vi "JitterDACADC.vi"() -> ()   [LabVIEW 2009]
uses:
  <vilib>/Analysis/4window.llb/windowTd.ctl
  <vilib>/measure/maspectr.llb/FFT Power Spectrum for 1 Chan.vi
  <vilib>/Analysis/2dsp.llb/Resample (constant to constant,single -channel).vi
  <vilib>/ptbypt/NI_PtbyPt.lvlib
  <vilib>/Analysis/NI_AALBase.lvlib
  <vilib>/Analysis/NI_AALPro.lvlib
  <vilib>/measure/NI_MAPro.lvlib
panel:
  in  "Clock RMS time jitter":dbl format="%#_6p"
  in  "Sampling Rate":dbl=3000000.0 format="%#_6p"
  out "df":dbl
  out "averages completed":dbl=20.0
  out "DAC / ADC Sampling Period":dbl format="%#_6p"
  out "Elapsed Time (Seconds)":dbl
  in  "averaging parameters":T1={"averaging mode"=enum."RMS averaging", "weighting mode"=enum."Exponential", "number of averages"=20} {"number of averages" min=1}
  in  "Test System\n AWGN noise (dBm)":dbl=-180.0 format="%#.6f"
  out "Power Spectrum of sampled signal":cluster{"f0":dbl, "df":dbl, "magnitude":dbl[]}(graph)={"f0"=0.0, "df"=5000.0, "magnitude"=[]}
  out "Time Domain of Sampled Signal":waveform(dbl)(graph)={"t0"=timestamp(0 s since 1904-01-01), "dt"=3.3333333333333335e-07, "Y"=[]}
  in  "Duration (Seconds)":dbl=0.0002 min=0.0 format="%#_6e"
  in  "Tone Power (dBm)":dbl format="%#.6f"
  in  "Tone Frequency":dbl=750000.0 min=0.0 max=1000000000.0 format="%#.6p"
  in  "DAC clock RMS time jitter":dbl=1e-09 min=0.0 format="%#_6p"
  # "DAC/ADC Demo"
  # "Sampling Rate of tone fed into zero order\nhold DAC (also rate at which ADC samples).\nMust be > 2 * Tone Frequency"
  # "Jittery output from ADC Bonus Question: \nWhat is the SNR of this signal for no jitter?"
  # "Clue: It isn't tone power / System AWGN noise power. \nConsider bandwidth."
  # "Test System ADC"
  # "df ~= 1 / duration"
  # "Hz / Bin"
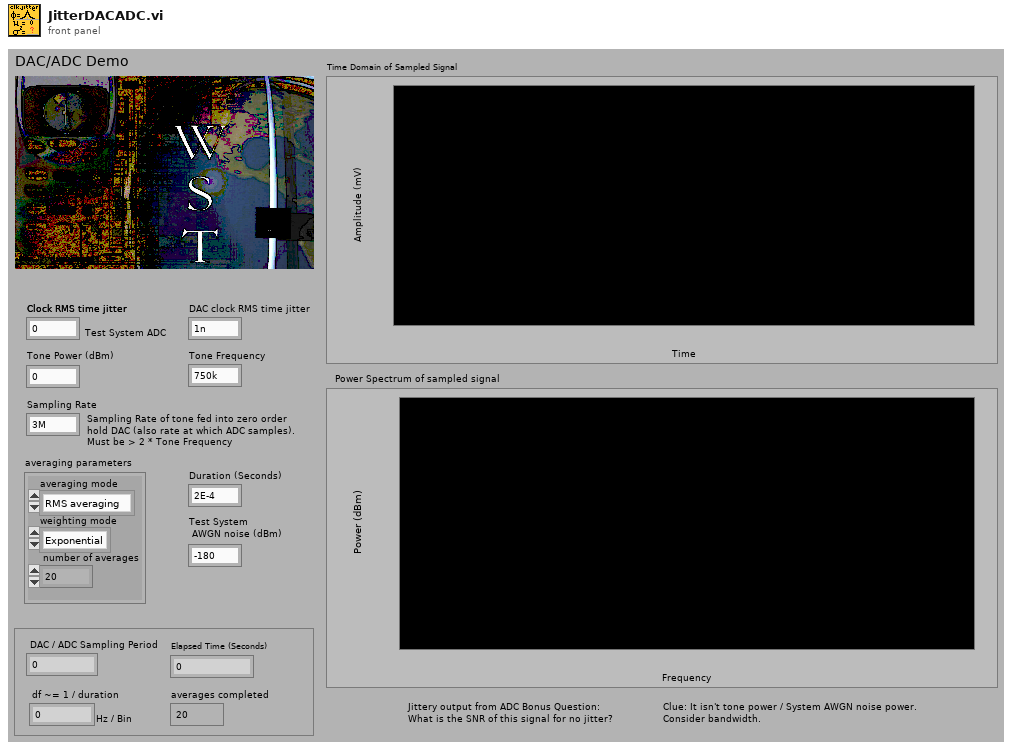
[diagram p1: front panel]
types:
  T1 = cluster{"averaging mode":enum16{"No averaging", "Vector averaging", "RMS averaging", "Peak hold"}, "weighting mode":enum16{"Linear", "Exponential"}, "number of averages":u32}
  T2 = typedef "NI_AALPro.lvlib/windowTd.ctl" = u32
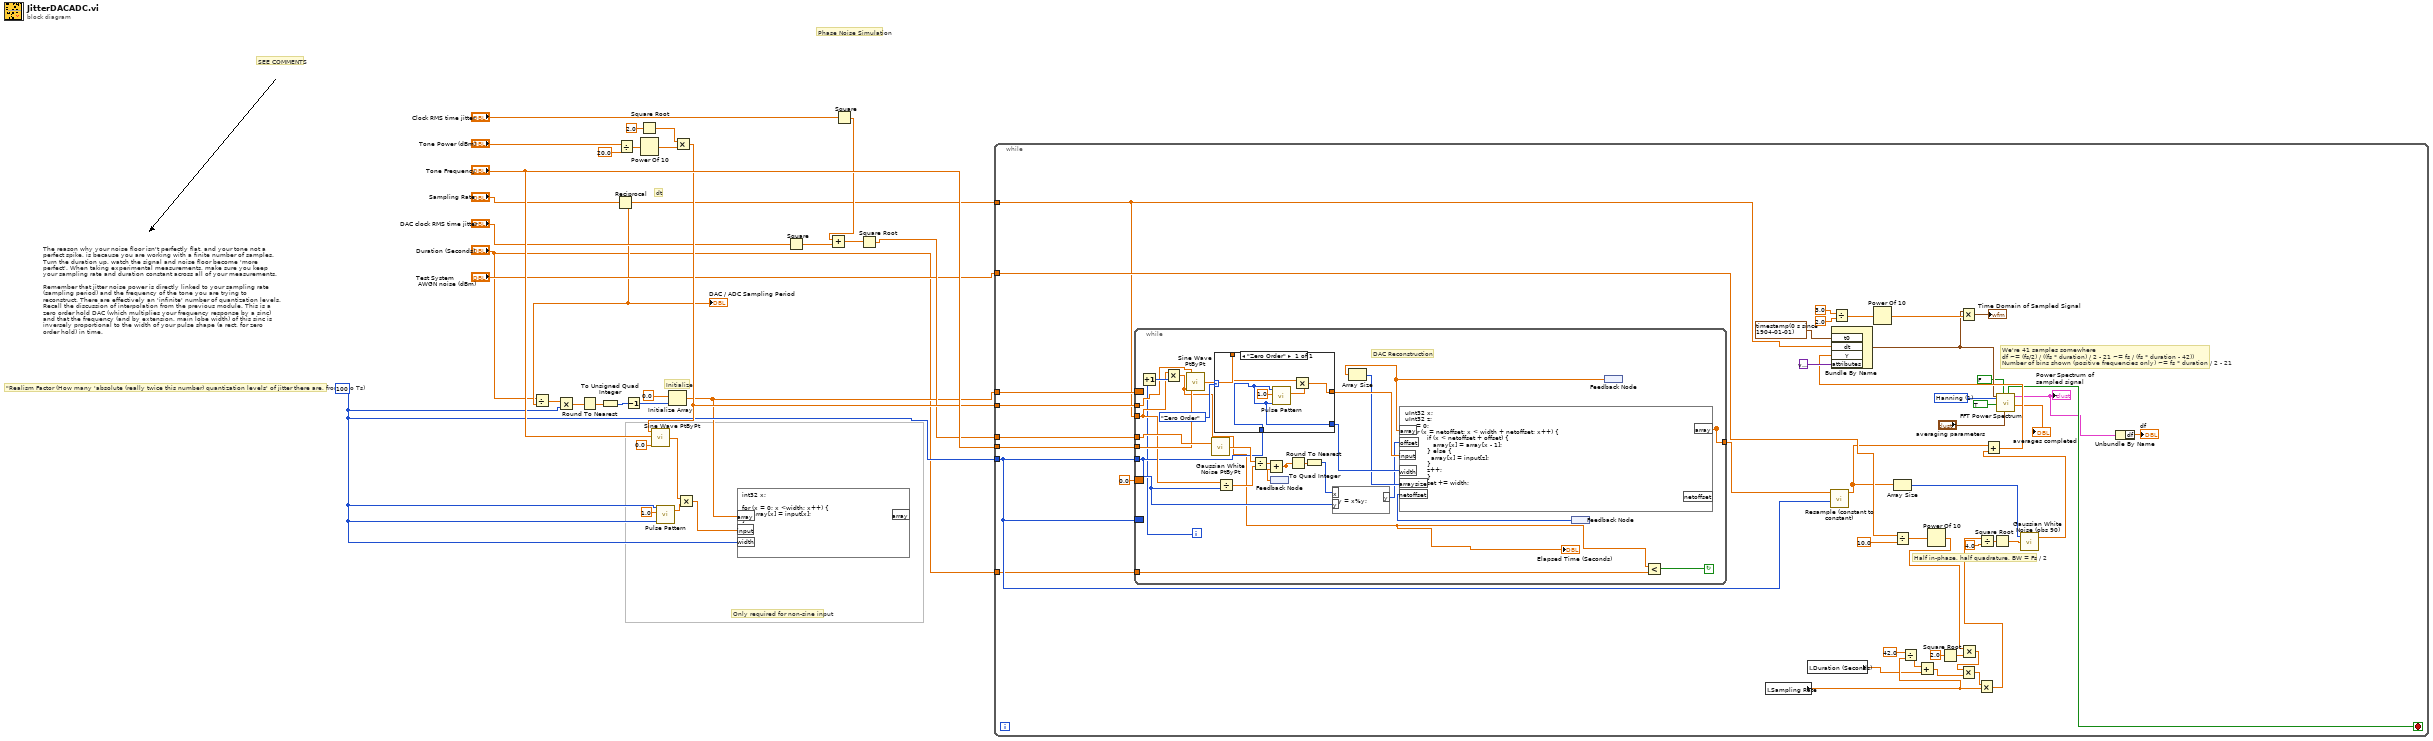
[diagram p0: block diagram]
diagram:
  w4 = 100
  # "SEE COMMENTS"
  # "The reason why your noise floor isn't perfectly flat, and your tone not a perfect spike, is because you are working with a finite number of samples. Turn the duration up, watch the signal and noise floor become 'more perfect'. When taking experimental measurements, make sure you keep your sampling rate and duration constant across all of your measurements.\n\nRemember that jitter noise power is directly linked to your sampling rate (sampling period) and the frequency of the tone you are trying to reconstruct. There are effectively an 'infinite' number of quantization levels. Recall the discussion of interpolation from the previous module. This is a zero order hold DAC (which multiplies your frequency response by a sinc) and that the frequency (and by extension, main lobe width) of this sinc is inversely proportional to the width of your pulse shape (a rect, for zero order hold) in time."
  # "Only required for non-sine input"
  # "\"Realism Factor (How many 'absolute (really twice this number) quantization levels' of jitter there are, from 0 to Ts)"
  # "Initialize"
  # "dt"
  # "Phase Noise Simulation"
  n1 = Reciprocal(x="Sampling Rate") -> (1/x=w5:dbl)
  "DAC / ADC Sampling Period" <- w5
  n2 = Divide(x="Duration (Seconds)", y=w5) -> (x/y=w21:dbl)
  n3 = Multiply(x=w21, y=w4) -> (x*y=w22:dbl)
  n4 = Round To Nearest(number=w22) -> (nearest integer value=w24:dbl)
  n5 = To Unsigned Quad Integer(1:w24) -> (0:w23:u64)
  n6 = Divide(x="Tone Power (dBm)", y=20.0) -> (x/y=w29:dbl)
  n7 = Decrement(x=w23) -> (x-1=w25:u64)
  n8 = Square Root(x=2.0) -> (sqrt(x)=w26:dbl)
  n9 = Power Of 10(x=w29) -> (10^x=w28:dbl)
  n10 = call <vilib>:"Pulse Pattern.vi"("width"=w4, "amplitude"=1.0, "samples"=w4) -> ("Pulse Pattern"=w15:dbl[])  [unwired: 1 in, 1 out]
  n11 = Initialize Array(0.0 ("element"), w25) -> (w2:dbl[])
  n12 = Multiply(x=w26, y=w28) -> (x*y=w18:dbl)
  n13 = call <vilib>:"Sine Wave PtByPt.vi"("time"=0.0, "frequency"="Tone Frequency", "amplitude"=w18) -> ("sine wave"=w13:dbl)  [unwired: 1 in]
  n14 = Multiply(x=w13, y=w15) -> (x*y=w14:dbl[])
  n15 = formula code="int32 x;\n\nfor (x = 0; x <width; x++) {\n     array[x] = input[x];\n}"("array"=w2, "input"=w14, "width"=w4) -> ()  [unwired: 1 out]
  n16 = Square(x="DAC clock RMS time jitter") -> (x^2=w11:dbl)
  n17 = Square(x="Clock RMS time jitter") -> (x^2=w10:dbl)
  n18 = Add(x=w10, y=w11) -> (x+y=w9:dbl)
  n19 = Square Root(x=w9) -> (sqrt(x)=w8:dbl)
  n20 = while {
    tunnel: "Tone Frequency" -> [w77]
    tunnel: w18 -> [w76]
    tunnel: w2 -> [w75]
    tunnel: w8 -> [w73]
    tunnel: "Test System\n AWGN noise (dBm)" -> [w66]
    tunnel: w5 -> [w60]
    tunnel: w4 -> [w52]
    tunnel: "Duration (Seconds)" -> [w38]
    stop <- w44 stop-if-true
    w59 = T2 1 items=["Rectangle"=0, "Hanning"=1, "Hamming"=2, "Blackman-Harris"=3, "Exact Blackman"=4, "Blackman"=5, "Flat Top"=6, "4 Term B-Harris "=7, "7 Term B-Harris"=8, "Low Sidelobe"=9, "Blackman Nuttall"=11, "Triangle"=30, "Kaiser"=60, "Dolph-Chebyshev"=61, "Gaussian"=62] ("window")
    # "We're 41 samples somewhere\ndf ~= (fs/2) / ((fs * duration) / 2 - 21 ~= fs / (fs * duration - 42))\nNumber of bins shown (positive frequencies only) ~= fs * duration / 2 - 21"
    # "Half in-phase, half quadrature, BW = Fs / 2"
    n21 = while {
      tunnel: w73 -> [w102]
      tunnel: w60 -> [w91]
      tunnel: w77 -> [w97]
      tunnel: w76 -> [w98]
      tunnel: w52 -> [w85]
      tunnel: [w89] -> w67
      tunnel: w38 -> [w80]
      border: w75 -> [_]
      border: w52 -> [_]
      border: 0.0 -> [_]
      i -> [w79]
      stop <- w104 continue-if-true
      # "DAC Reconstruction"
      n22 = Increment(x=w79) -> (x+1=w99:i32)
      n23 = Multiply(x=w91, y=w99) -> (x*y=w78:dbl)
      "Elapsed Time (Seconds)" <- w78
      n24 = call <vilib>:"Sine Wave PtByPt.vi"("time"=w78, "frequency"=w97, "amplitude"=w98) -> ("sine wave"=w103:dbl)  [unwired: 1 in]
      n25 = call <vilib>:"Gaussian White Noise PtByPt.vi"("standard deviation"=w102) -> ("Gaussian white noise"=w92:dbl)  [unwired: 2 in]
      n26 = case shown="\"Zero Order\"" enum16{"Zero Order"}."Zero Order" ("DAC Interpolation type") {
        tunnel: w85 -> [w105]
        tunnel: w103 -> [w107]
        tunnel: [w106] -> w101
        tunnel: [w105] -> w100
        frame "Zero Order" {
          n27 = call <vilib>:"Pulse Pattern.vi"("width"=w105, "amplitude"=1.0, "samples"=w105) -> ("Pulse Pattern"=w108:dbl[])  [unwired: 1 in, 1 out]
          n28 = Multiply(x=w107, y=w108) -> (x*y=w106:dbl[])
        }
      }
      n29 = Divide(x=w91, y=w85) -> (x/y=w93:dbl)
      n30 = Divide(x=w92, y=w93) -> (x/y=w83:dbl)
      n31 = feedback #1() -> (w82:dbl)
      n32 = Add(x=w83, y=w82) -> (x+y=w81:dbl)
      n33 = Round To Nearest(number=w81) -> (nearest integer value=w84:dbl)
      n34 = To Quad Integer(1:w84) -> (0:w87:i64)
      n35 = formula code="y = x%y;"("x"=w87, "y"=w85) -> ("y"=w86:i32)
      n36 = feedback #2() -> (w95:i32)
      n37 = feedback #3() -> (w90:dbl[])
      n38 = Array Size(array=w90) -> (size(s)=w94:i32)
      n39 = formula code="uInt32 x;\nuInt32 z;\n   z = 0;\n   for (x = netoffset; x < width + netoffset; x++) {\n           if (x < netoffset + offset) {\n              array[x] = array[x - 1];\n           } else {\n             array[x] = input[z];\n           }\n           z++;\n           }\n  netoffset += width;"("array"=w90, "offset"=w86, "input"=w101, "width"=w100, "netoffset"=w95, "arraysize"=w94) -> ("array"=w89:dbl[], "netoffset"=w96:i32)
      n40 = Less?(x=w78, y=w80) -> (x < y?=w104:bool)
    }
    n41 = local read "Sampling Rate"() -> (w36:dbl)
    n42 = local read "Duration (Seconds)"() -> (w34:dbl)
    n43 = call-poly <vilib>:"Resample (constant to constant).vi"("dt"=w52, "X"=w67) -> ("Y"=w56:dbl[])  [unwired: 7 in, 2 out]
    n44 = Divide(x=3.0, y=2.0) -> (x/y=w70:dbl)
    n45 = Power Of 10(x=w70) -> (10^x=w68:dbl)
    n46 = Array Size(array=w56) -> (size(s)=w57:i32)
    n47 = Divide(x=w66, y=10.0) -> (x/y=w64:dbl)
    n48 = Divide(x=42.0, y=w36) -> (x/y=w35:dbl)
    n49 = Add(x=w35, y=w34) -> (x+y=w33:dbl)
    n50 = Power Of 10(x=w64) -> (10^x=w47:dbl)
    n51 = Square Root(x=2.0) -> (sqrt(x)=w50:dbl)
    n52 = Multiply(x=w47, y=w50) -> (x*y=w49:dbl)
    n53 = Multiply(x=w49, y=w33) -> (x*y=w48:dbl)
    n54 = Multiply(x=w48, y=w36) -> (x*y=w46:dbl)
    n55 = Divide(x=w46, y=4.0) -> (x/y=w61:dbl)
    n56 = Square Root(x=w61) -> (sqrt(x)=w62:dbl)
    n57 = call <vilib>:"Gaussian White Noise (obs 90).vi"("standard deviation"=w62, "samples"=w57) -> ("Gaussian noise pattern"=w45:dbl[])  [unwired: 1 in, 1 out]
    n58 = Add(x=w56, y=w45) -> (x+y=w55:dbl[])
    n59 = Bundle By Name("t0"=timestamp(0 s since 1904-01-01), "dt"=w60, "Y"=w55, "attributes"=variant) -> (w53:waveform(dbl))  [unwired: 1 in]
    n60 = Multiply(x=w53, y=w68) -> (x*y=→"Time Domain of Sampled Signal":waveform(dbl))
    n61 = call-poly <vilib>:"FFT Power Spectrum.vi"("averaging parameters"="averaging parameters", "restart averaging (F)"=FALSE, "dB On (F)"=TRUE, "window"=w59, "time signal"=w53) -> ("averages completed"=→"averages completed":dbl, "power spectrum"=w40:cluster{"f0":dbl, "df":dbl, "magnitude":dbl[]}, "averaging done"=w44:bool)  [unwired: 3 in, 1 out]
    "Power Spectrum of sampled signal" <- w40
    n62 = Unbundle By Name(w40) -> ("df"=→"df":dbl)
  }
